vi "Maxi Gauge-Get Set Point Status.vi"(0 "VISA-Ressource in":refnum<visa-resource-name>, 1 "Node address":i8=-1 min=-1 max=31 step=1, 5 "Fehler (Eingang)":errorcluster) -> (12 "Relay A":u8(ring)=3 items=["off", "on"], 13 "Relay F":u8(ring)=3 items=["off", "on"], 14 "VISA-Ressource out":refnum<visa-resource-name>, 15 "Relay B":u8(ring)=3 items=["off", "on"], 16 "Relay C":u8(ring)=3 items=["off", "on"], 17 "Relay D":u8(ring)=3 items=["off", "on"], 18 "Relay E":u8(ring)=3 items=["off", "on"], 19 "Fehler (Ausgang)":errorcluster)   [LabVIEW 2013, in "Maxi Gauge.lvlib"]
uses:
  <instrlib>/Maxi Gauge/Maxi Gauge.lvlib
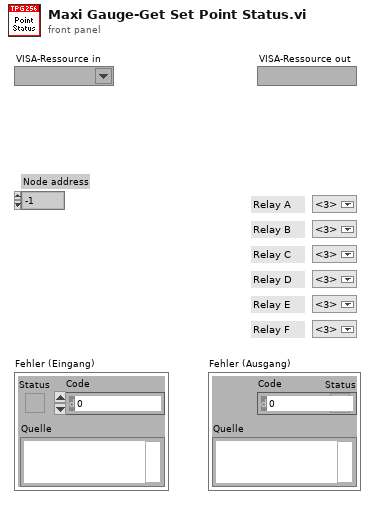
[diagram p1: front panel]
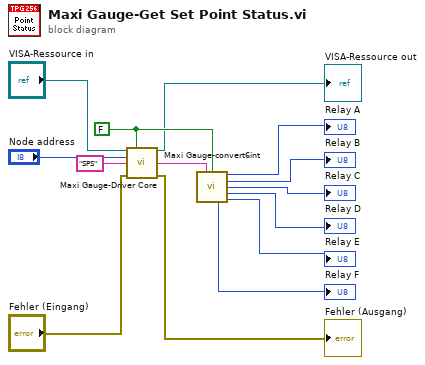
[diagram p0: block diagram]
diagram:
  w5 = FALSE ("Write/Read")
  n1 = call <instrlib>:"Maxi Gauge-Driver Core.vi"("VISA-Ressource in"="VISA-Ressource in", "Write/Read"=w5, "Node address"="Node address", "Command"="SPS", "Fehler (Eingang)"="Fehler (Eingang)") -> ("VISA-Ressource out"=→"VISA-Ressource out":refnum<visa-resource-name>, "String Out"=w7:string, "Fehler (Ausgang)"=→"Fehler (Ausgang)":errorcluster)  [unwired: 8 in]
  n2 = call <instrlib>:"Maxi Gauge-convert6int.vi"("String in"=w7, "W/R [W: Int in; Str out ]"=w5) -> ("Integer1 out"=→"Relay A":u8, "Integer2 out"=→"Relay B":u8, "Integer3 out"=→"Relay C":u8, "Integer4 out"=→"Relay D":u8, "Integer6 out"=→"Relay F":u8, "Integer5 out"=→"Relay E":u8)  [unwired: 7 in, 1 out]
